vi "FisherPaykel Set Sense Profile.vi"(7 "Debug":bool, 8 "Error In":errorcluster, 9 "Set Sense Profile":T2, 10 "Main Command":T1=">SNS", 11 "VISA Refnum in":refnum<visa-resource-name>) -> (0 "Error Out":errorcluster, 2 "Command (Debug)":string, 3 "VISA Refnum out":refnum<visa-resource-name>)   [LabVIEW 2016]
uses:
  Type Definitions/FisherPaykel Set Sense Profile.ctl
  Type Definitions/Fisher Paykel Main Command.ctl
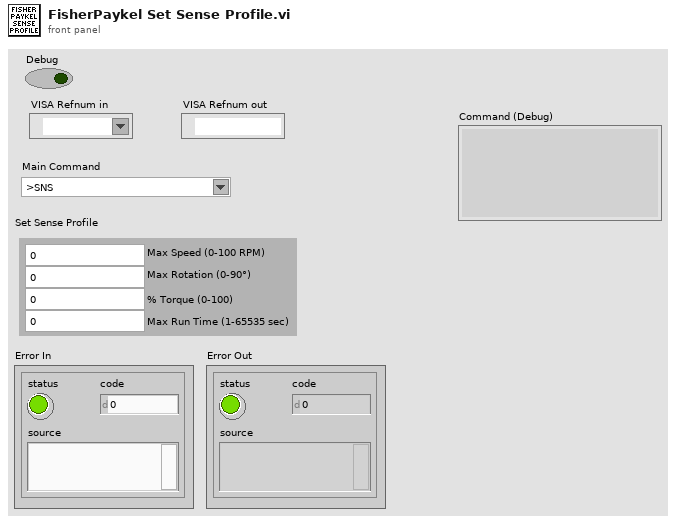
[diagram p1: front panel]
types:
  T1 = typedef "Fisher Paykel Main Command.ctl" = string
  T2 = typedef "FisherPaykel Set Sense Profile.ctl" = cluster{"Max Speed (0-100 RPM)":u16, "Max Rotation (0-90°)":u16, "% Torque (0-100)":u16, "Max Run Time (1-65535 sec)":u16}
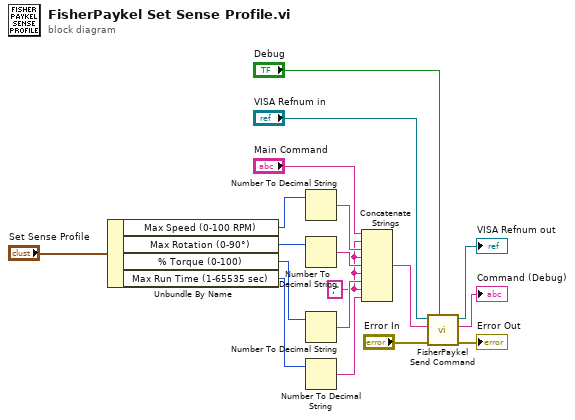
[diagram p0: block diagram]
diagram:
  w2 = ","
  n1 = Unbundle By Name("Set Sense Profile") -> ("Max Speed (0-100 RPM)"=w9:u16, "Max Rotation (0-90°)"=w8:u16, "% Torque (0-100)"=w7:u16, "Max Run Time (1-65535 sec)"=w6:u16)
  n2 = Number To Decimal String(number=w9) -> (decimal integer string=w5:string)  [unwired: 1 in]
  n3 = Number To Decimal String(number=w8) -> (decimal integer string=w4:string)  [unwired: 1 in]
  n4 = Number To Decimal String(number=w7) -> (decimal integer string=w3:string)  [unwired: 1 in]
  n5 = Number To Decimal String(number=w6) -> (decimal integer string=w1:string)  [unwired: 1 in]
  n6 = Concatenate Strings("Main Command", w2, w5, w2, w4, w2, w3, w2, w1) -> (w17:string)
  n7 = call "FisherPaykel Send Command.vi"("Debug"="Debug", "error in (no error)"="Error In", "Send Command"=w17, "VISA Refnum in"="VISA Refnum in") -> ("error out"=→"Error Out":errorcluster, "Command (Debug)"=→"Command (Debug)":string, "VISA Refnum out"=→"VISA Refnum out":refnum<visa-resource-name>)  [unwired: 5 in]
